vi "Default.vi"(8 "error in (no error)":errorcluster, 11 "CallVIStep in":refnum<class "CallVIStep.lvclass">) -> (0 "error out":errorcluster, 3 "CallVIStep out":refnum<class "CallVIStep.lvclass">)   [LabVIEW 2015, in "CallVIStep.lvclass"]
uses:
  CallVIStep.lvclass
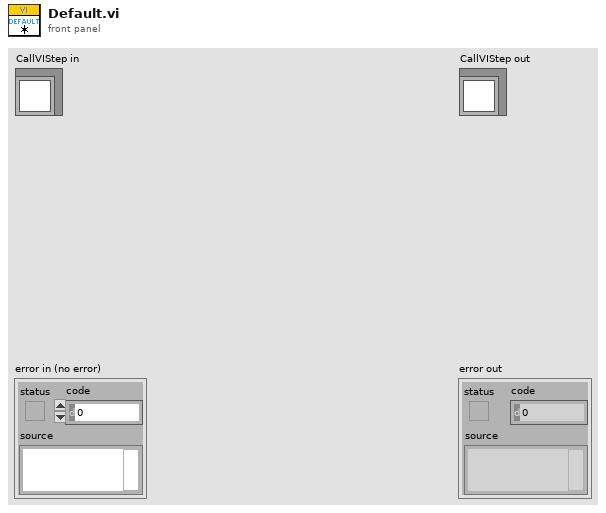
[diagram p1: front panel]
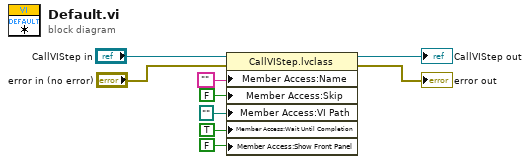
[diagram p0: block diagram]
diagram:
  n1 = property class="CallVIStep.lvclass"(reference="CallVIStep in", error in="error in (no error)", "Member Access:Name"="", "Member Access:Skip"=FALSE ("Skip"), "Member Access:VI Path"=path "", "Member Access:Wait Until Completion"=TRUE ("Skip"), "Member Access:Show Front Panel"=FALSE ("Show Front Panel")) -> (reference out=→"CallVIStep out":refnum<class "CallVIStep.lvclass">, error out=→"error out":errorcluster)
